vi "Register Callbacks.vi"(8 "error in (no error)":errorcluster, 11 "Tree Alias":T1) -> (0 "error out":errorcluster, 2 "Callbacks":T2, 3 "Tree Alias dup":T1)   [LabVIEW 2020, in "NI_VS UI Tree Alias Browser.lvlib"]
uses:
  <vilib>/NI VeriStand/UI Controls/Tree and Alias Browser/NI_VS UI Tree Alias Browser.lvlib
  <vilib>/NI VeriStand/UI Controls/Tree and Alias Browser/Tree Alias Browser Ref.ctl
  NationalInstruments.VeriStand.SystemStorageUI
  <vilib>/NI VeriStand/UI Controls/Tree and Alias Browser/Callback Type.ctl
  <vilib>/NI VeriStand/UI Controls/Tree and Alias Browser/Net Event Data Ref.ctl
  <vilib>/NI VeriStand/UI Controls/Tree and Alias Browser/Net Event Data.ctl
  <vilib>/NI VeriStand/UI Controls/Tree and Alias Browser/Net Event.ctl
  <vilib>/NI VeriStand/UI Controls/Tree and Alias Browser/Dbl Click Callback.vi
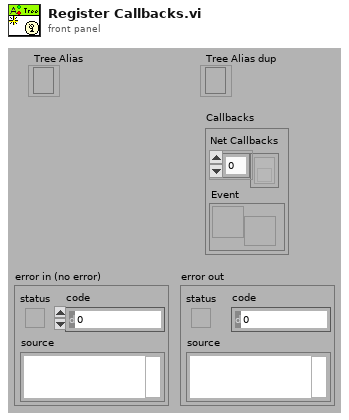
[diagram p1: front panel]
types:
  T1 = typedef "NI_VS UI Tree Alias Browser.lvlib/Tree Alias Browser Ref.ctl" = refnum<k24>
  T2 = typedef "NI_VS UI Tree Alias Browser.lvlib/Callback Type.ctl" = cluster{"Net Callbacks":refnum<k27>[], "Event":T3}
  T3 = typedef "NI_VS UI Tree Alias Browser.lvlib/Net Event Data Ref.ctl" = refnum<user-event>
  T4 = typedef "NI_VS UI Tree Alias Browser.lvlib/Net Event Data.ctl" = cluster{"Type":T5, "Data":variant}
  T5 = typedef "NI_VS UI Tree Alias Browser.lvlib/Net Event.ctl" = enum16{"SelectedItem", "DblClick"}
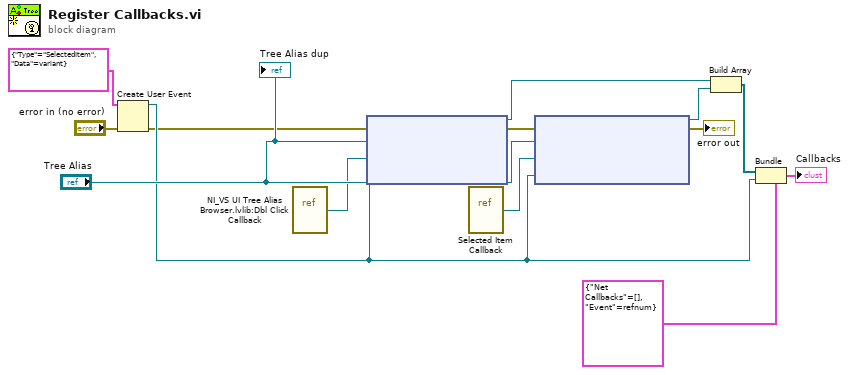
[diagram p0: block diagram]
diagram:
  n1 = Create User Event(user event datatype=T4 {"Type"=enum."SelectedItem", "Data"=variant} ("Net Event Data"), error in="error in (no error)") -> (user event=w5:refnum<user-event>, error out=w2:errorcluster)
  n2 = vi-ref "NI_VS UI Tree Alias Browser.lvlib:Dbl Click Callback.vi"() -> ("vi reference"=w1:refnum<vi>)
  n3 = node(w2, "Tree Alias", w1, w5) -> (w12:refnum<k27>, w11:errorcluster)  [unwired: 1 in]
  n4 = vi-ref <vilib>:"Selected Item Callback.vi"() -> ("vi reference"=w10:refnum<vi>)
  n5 = node(w11, "Tree Alias", w10, w5) -> (w13:refnum<k27>, →"error out":errorcluster)  [unwired: 1 in]
  n6 = Build Array(w12, w13) -> (w6:refnum<k27>[])
  n7 = Bundle(cluster=T2 {"Net Callbacks"=[], "Event"=refnum} ("Callback"), "Net Callbacks"=w6, "Event"=w5) -> (→"Callbacks":T2)
  "Tree Alias dup" <- "Tree Alias"
